vi "PCE-Connect.vi"(0 "IP":string="132.204.60.164", 7 "Port":u16=8080) -> (4 "connection ID":refnum<k5>, 15 "error out":errorcluster)   [LabVIEW 2011]
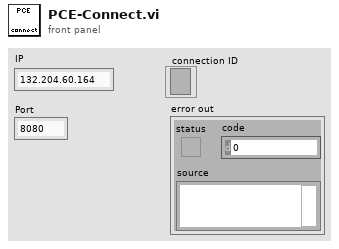
[diagram p1: front panel]
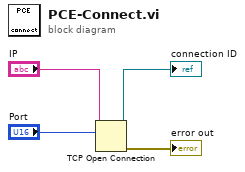
[diagram p0: block diagram]
diagram:
  n1 = TCP Open Connection(address="IP", remote port or service name="Port") -> (connection ID=→"connection ID":refnum<k5>, error out=→"error out":errorcluster)  [unwired: 3 in]
